vi "Scan  Barcode.vi"(3 "±ø½X¦ì¼Æ":i32=6, 4 "前面板窗口:标题":string="条码输入...", 5 "no check?":bool) -> (0 "SN":string, 1 "P/F":bool)   [LabVIEW 2018]
panel:
  in  "Cancel 2":bool
  in  "OK":bool
  in  "Barcode":string
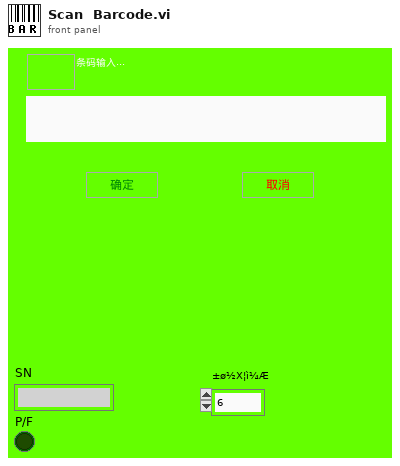
[diagram p1: front panel]
types:
  T1 = enum32{"Invalid", "Standard", "Closed", "Hidden", "Minimized", "Maximized"}
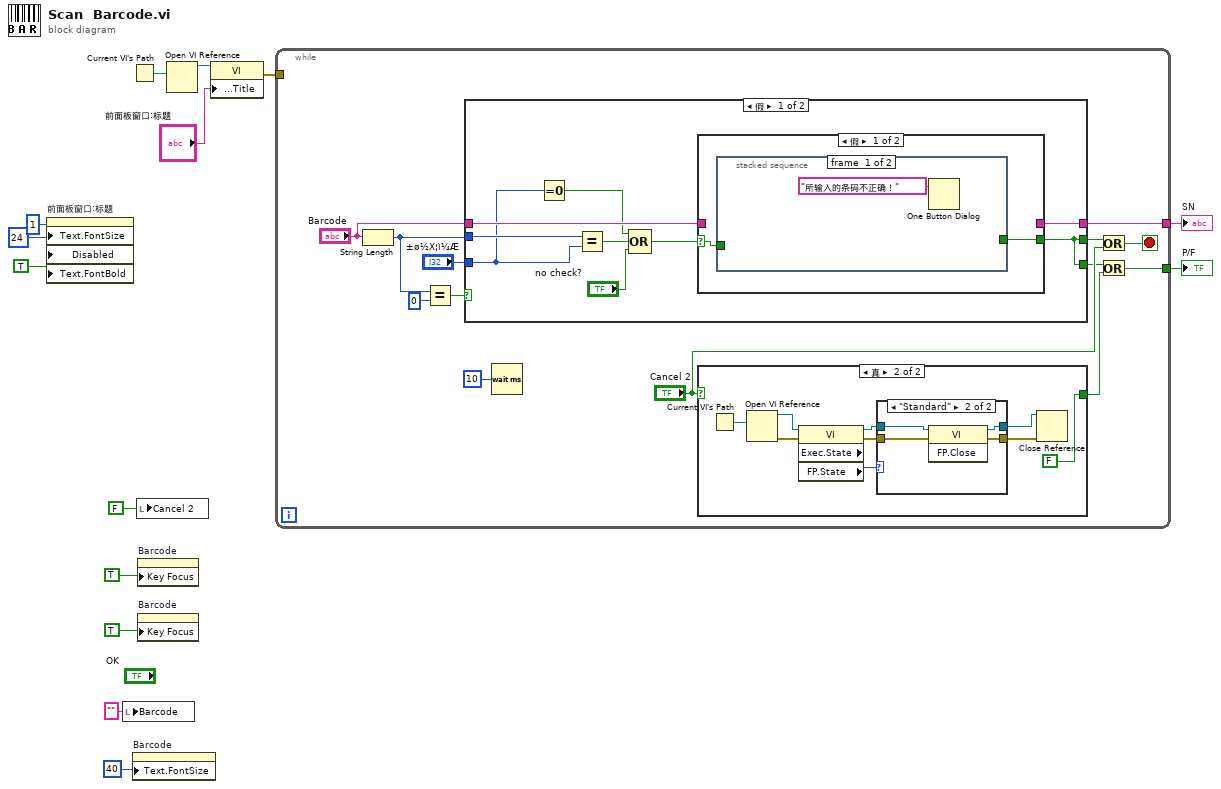
[diagram p0: block diagram]
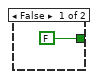
[diagram p2: hidden frame]
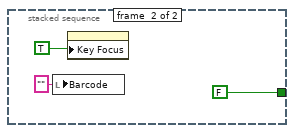
[diagram p4: hidden frame]
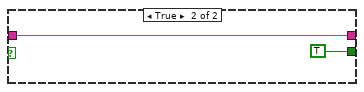
[diagram p5: hidden frame]
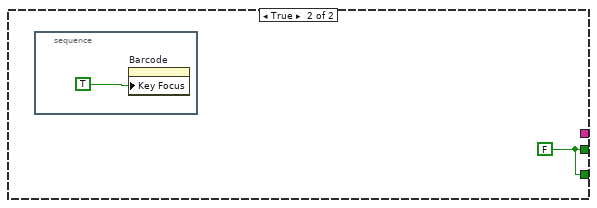
[diagram p6: hidden frame]
diagram:
  n1 = property on="前面板窗口:标题" class="Str"("Text.FontSize"=u32 24 ("文本.字体:字号"), "Disabled"=u8 1 ("禁用"), "Text.FontBold"=TRUE ("文本.字体:粗体")) -> ()  [unwired: 2 in, 2 out]
  n2 = local write "Barcode"("" ("Barcode")) -> ()
  n3 = Current VI's Path() -> (path=w13:path)
  n4 = property on="Barcode" class="Str"("Text.FontSize"=u32 40 ("Text.Font:Size")) -> ()  [unwired: 2 in, 2 out]
  n5 = local write "Cancel 2"(FALSE ("Cancel 2")) -> ()
  n6 = property on="Barcode" class="Str"("Key Focus"=TRUE) -> ()  [unwired: 2 in, 2 out]
  n7 = property on="Barcode" class="Str"("Key Focus"=TRUE) -> ()  [unwired: 2 in, 2 out]
  n8 = Open VI Reference(vi path=w13) -> (vi reference=w12:refnum<vi>)  [unwired: 2 in, 4 out]
  n9 = property class="VI"(reference=w12, "Front Panel.Title"="前面板窗口:标题") -> (error out=w5:errorcluster)  [unwired: 1 in, 1 out]
  n10 = while {
    tunnel: [w16] -> w6
    tunnel: [w19] -> w7
    tunnel: w5 -> [_]
    stop <- w23 stop-if-true
    n11 = String Length(string="Barcode") -> (length=w24:i32)
    n12 = Equal?(x=w24, y=0) -> (x = y?=w25:bool)
    n13 = case shown="假" w25 {
      tunnel: w24 -> [w49 _]
      tunnel: [w47 w59] -> w22
      tunnel: "Barcode" -> [w48 _]
      tunnel: "±ø½X¦ì¼Æ" -> [w43 _]
      tunnel: [w47 w59] -> w17
      tunnel: [w46 _] -> w19
      frame False {
        n14 = Equal To 0?(x=w43) -> (x = 0?=w42:bool)
        n15 = Equal?(x=w49, y=w43) -> (x = y?=w50:bool)
        n16 = Compound Arithmetic op=OR(w42, w50, "no check?") -> (w45:bool)
        n17 = case shown="假" w45 {
          selector: w45 -> [w52 _]
          tunnel: [w51 TRUE] -> w47
          tunnel: w48 -> [_ w57]
          tunnel: [_ w57] -> w46
          frame False {
            n18 = stacked-sequence {
              tunnel: w52 -> [_ _]
              tunnel: [_ FALSE] -> w51
              frame #0 {
                n19 = One Button Dialog(message="所输入的条码不正确！" ("消息")) -> ()  [unwired: 2 out]
              }
              frame #1 {
                n20 = local write "Barcode"("" ("Barcode")) -> ()
                n21 = property on="Barcode" class="Str"("Key Focus"=TRUE) -> ()  [unwired: 2 in, 2 out]
              }
            }
          }
          frame True {
          }
        }
      }
      frame True {
        w59 = FALSE
        n22 = stacked-sequence {
          frame #0 {
            n23 = property on="Barcode" class="Str"("Key Focus"=TRUE) -> ()  [unwired: 2 in, 2 out]
          }
        }
      }
    }
    n24 = Wait (ms)(milliseconds to wait=u32 10) -> ()  [unwired: 1 out]
    n25 = case shown="真" "Cancel 2" {
      tunnel: [FALSE FALSE] -> w15
      frame False {
      }
      frame True {
        n26 = Current VI's Path() -> (path=w37:path)
        n27 = Open VI Reference(vi path=w37) -> (vi reference=w35:refnum<vi>, error out=w36:errorcluster)  [unwired: 2 in, 3 out]
        n28 = property class="VI" props=["Exec.State", "FP.State"](reference=w35, error in=w36) -> (reference out=w31:refnum<vi>, error out=w30:errorcluster, "FP.State"=w32:T1)  [unwired: 1 out]
        n29 = case shown="\"Standard\"" w32 {
          tunnel: w30 -> [_ w41]
          tunnel: w31 -> [_ w40]
          tunnel: [_ w39] -> w33
          tunnel: [_ w38] -> w34
          frame "Invalid", Default {
          }
          frame "Standard" {
            n30 = invoke class="VI" method="FP.Close"(reference=w40, error in=w41) -> (reference out=w38:refnum<vi>, error out=w39:errorcluster)  [unwired: 1 in, 1 out]
          }
        }
        n31 = Close Reference(reference=w34, error in (no error)=w33) -> ()  [unwired: 1 out]
      }
    }
    n32 = Or(x=w22, y="Cancel 2") -> (x .or. y?=w23:bool)
    n33 = Or(x=w17, y=w15) -> (x .or. y?=w16:bool)
  }
  "SN" <- w7
  "P/F" <- w6
